vi "LEDcst.vi"() -> (3 "Lights Values":T1)   [LabVIEW 2014]
uses:
  LEDdriver/LEDPorts.ctl
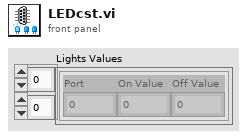
[diagram p1: front panel]
types:
  T1 = typedef "LEDPorts.ctl" = cluster{"Port":i16, "On Value":u8, "Off Value":u8}[][]
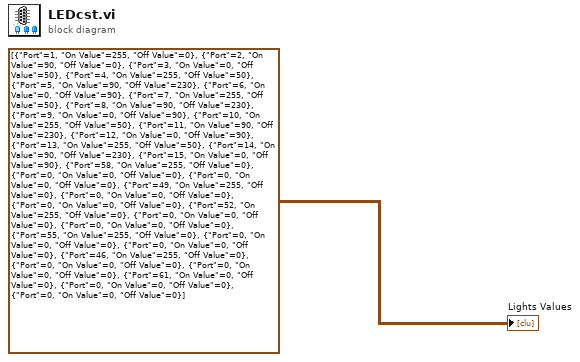
[diagram p0: block diagram]
diagram:
  "Lights Values" <- T1 [[{"Port"=1, "On Value"=255, "Off Value"=0}, {"Port"=2, "On Value"=90, "Off Value"=0}, {"Port"=3, "On Value"=0, "Off Value"=50}], [{"Port"=4, "On Value"=255, "Off Value"=50}, {"Port"=5, "On Value"=90, "Off Value"=230}, {"Port"=6, "On Value"=0, "Off Value"=90}], [{"Port"=7, "On Value"=255, "Off Value"=50}, {"Port"=8, "On Value"=90, "Off Value"=230}, {"Port"=9, "On Value"=0, "Off Value"=90}], [{"Port"=10, "On Value"=255, "Off Value"=50}, {"Port"=11, "On Value"=90, "Off Value"=230}, {"Port"=12, "On Value"=0, "Off Value"=90}], [{"Port"=13, "On Value"=255, "Off Value"=50}, {"Port"=14, "On Value"=90, "Off Value"=230}, {"Port"=15, "On Value"=0, "Off Value"=90}], [{"Port"=58, "On Value"=255, "Off Value"=0}, {"Port"=0, "On Value"=0, "Off Value"=0}, {"Port"=0, "On Value"=0, "Off Value"=0}], [{"Port"=49, "On Value"=255, "Off Value"=0}, {"Port"=0, "On Value"=0, "Off Value"=0}, {"Port"=0, "On Value"=0, "Off Value"=0}], [{"Port"=52, "On Value"=255, "Off Value"=0}, {"Port"=0, "On Value"=0, "Off Value"=0}, {"Port"=0, "On Value"=0, "Off Value"=0}], [{"Port"=55, "On Value"=255, "Off Value"=0}, {"Port"=0, "On Value"=0, "Off Value"=0}, {"Port"=0, "On Value"=0, "Off Value"=0}], [{"Port"=46, "On Value"=255, "Off Value"=0}, {"Port"=0, "On Value"=0, "Off Value"=0}, {"Port"=0, "On Value"=0, "Off Value"=0}], [{"Port"=61, "On Value"=0, "Off Value"=0}, {"Port"=0, "On Value"=0, "Off Value"=0}, {"Port"=0, "On Value"=0, "Off Value"=0}]] ("Lights Values")
